vi "Read Stop State.vi"(8 "error in (no error)":errorcluster, 11 "StopEnabledActor in":refnum<class "StopEnabledActor.lvclass">) -> (0 "error out":errorcluster, 2 "Stop?":bool, 3 "StopEnabledActor out":refnum<class "StopEnabledActor.lvclass">)   [LabVIEW 2017, in "StopEnabledActor.lvclass"]
uses:
  StopEnabledActor.lvclass
  StopEnabledActor.lvclass/StopEnabledActor.ctl
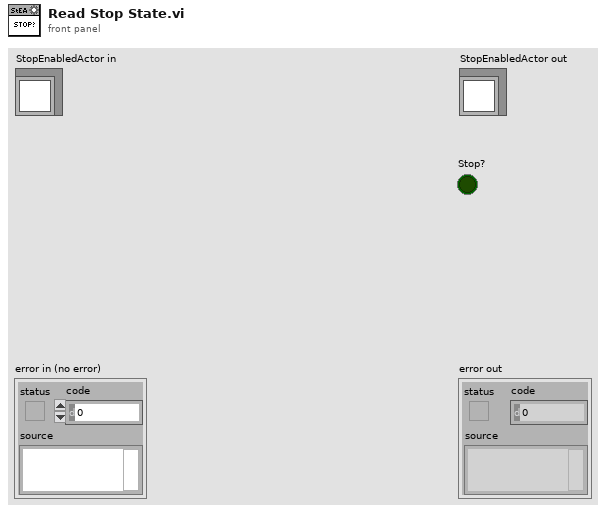
[diagram p1: front panel]
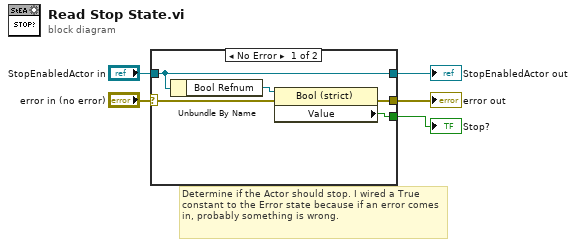
[diagram p0: block diagram]
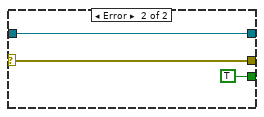
[diagram p2: hidden frame]
diagram:
  # "Determine if the Actor should stop. I wired a True constant to the Error state because if an error comes in, probably something is wrong."
  n1 = case shown="No Error" "error in (no error)" {
    selector: "error in (no error)" -> [w9 w13]
    tunnel: [w8 w13] -> w4
    tunnel: [w10 w12] -> w2
    tunnel: "StopEnabledActor in" -> [w10 w12]
    tunnel: [w6 TRUE] -> w1
    frame No Error {
      n2 = Unbundle By Name(w10) -> ("Bool Refnum"=w7:refnum<vi>)
      n3 = property class="Bool (strict)"(reference=w7, error in=w9) -> (error out=w8:errorcluster, "Value"=w6:bool)  [unwired: 1 out]
    }
    frame Error {
    }
  }
  "error out" <- w4
  "StopEnabledActor out" <- w2
  "Stop?" <- w1
